vi "MeasureTransconductance.vi"(0 ".NET Refnum in":refnum<k24>, 1 "UiDefinition":T1, 2 "Junction Name":string, 5 ".NET Refnum":refnum<k24>, 7 "appended path":path, 9 "Path":path, 12 "new file path (Not A Path if cancelled)":path, 13 "Function":string) -> (4 "Cluster":cluster{dbl[], dbl[]}, 15 "error out":errorcluster)   [LabVIEW 2020]
uses:
  UIReferences.ctl
  C:/Users/User/Desktop/Automation/CurrentVersion/LabviewDXFViewer/bin/Release/LabviewDXFViewer.exe
  LabviewDXFViewer/bin/Release/LabviewDXFViewer.exe
  <vilib>/Utility/file.llb/Write Delimited Spreadsheet (DBL).vi
  <vilib>/Utility/file.llb/Write Delimited Spreadsheet (string).vi
panel:
  in  "CurrentPositionIndex":i32
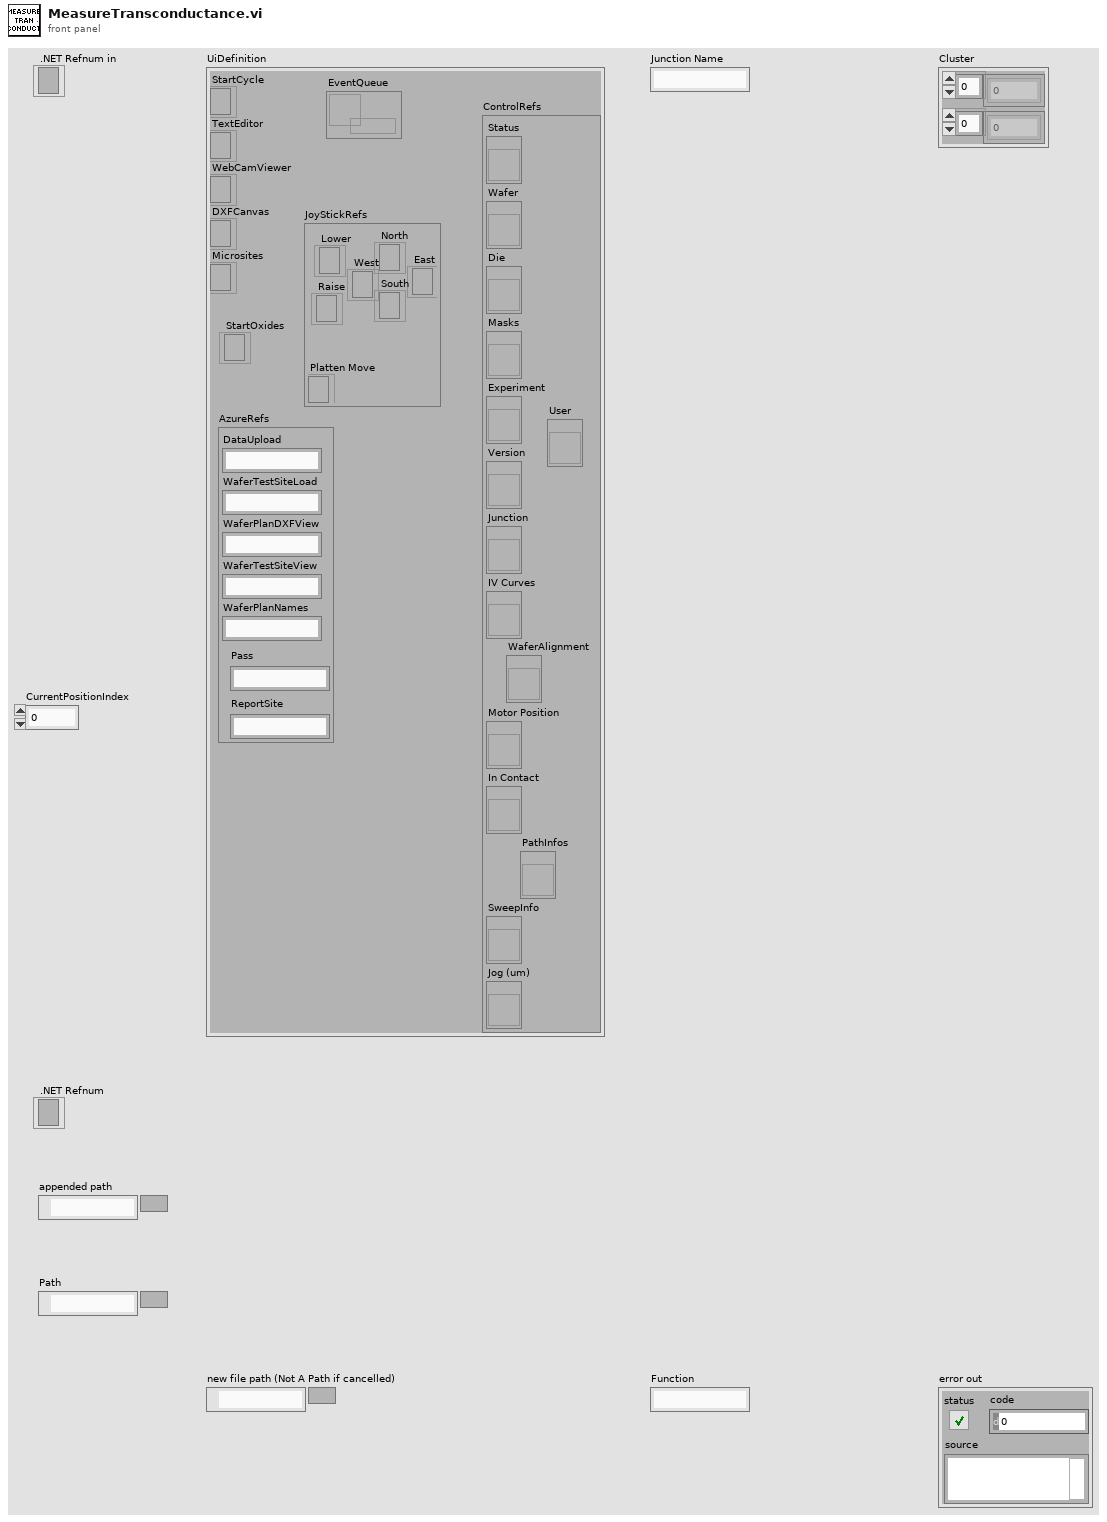
[diagram p1: front panel]
types:
  T1 = typedef "UIReferences.ctl" = cluster{"StartCycle":refnum<k24>, "TextEditor":refnum<k24>, "WebCamViewer":refnum<k24>, "DXFCanvas":refnum<k24>, "Microsites":refnum<k24>, "JoyStickRefs":cluster{"North":refnum<k24>, "Lower":refnum<k24>, "Raise":refnum<k24>, "Platten Move":refnum<k24>, "West":refnum<k24>, "East":refnum<k24>, "South":refnum<k24>}, "AzureRefs":cluster{"DataUpload":string, "WaferTestSiteLoad":string, "WaferPlanDXFView":string, "WaferTestSiteView":string, "WaferPlanNames":string, "Pass":string, "ReportSite":string}, "ControlRefs":cluster{"Status":refnum<vi>, "Wafer":refnum<vi>, "Die":refnum<vi>, "Masks":refnum<vi>, "Experiment":refnum<vi>, "Version":refnum<vi>, "Junction":refnum<vi>, "IV Curves":refnum<vi>, "Motor Position":refnum<vi>, "In Contact":refnum<vi>, "SweepInfo":refnum<vi>, "Jog (um)":refnum<vi>, "PathInfos":refnum<vi>, "User":refnum<vi>, "WaferAlignment":refnum<vi>}, "EventQueue":refnum<queue>, "StartOxides":refnum<k24>}
  T2 = typedef "CapacitanceInfos.ctl" = cluster{"Conductance":dbl, "CapacitanceIV":dbl, "Intercept":dbl, "CapacitanceSW":dbl, "Sum":dbl, "CapacitanceInfos":T3[], "CapacitancePhase":dbl, "dC/dV":dbl, "Function":string, "OtherInfo":dbl[][]}
  T3 = typedef "CapacitanceRecord.ctl" = cluster{"Freq":dbl, "Vpp":dbl, "PhaseS":dbl, "Irms":dbl, "PhaseC":dbl, "Theta":dbl, "VDrive":dbl, "Capacitance":dbl, "Other":dbl}
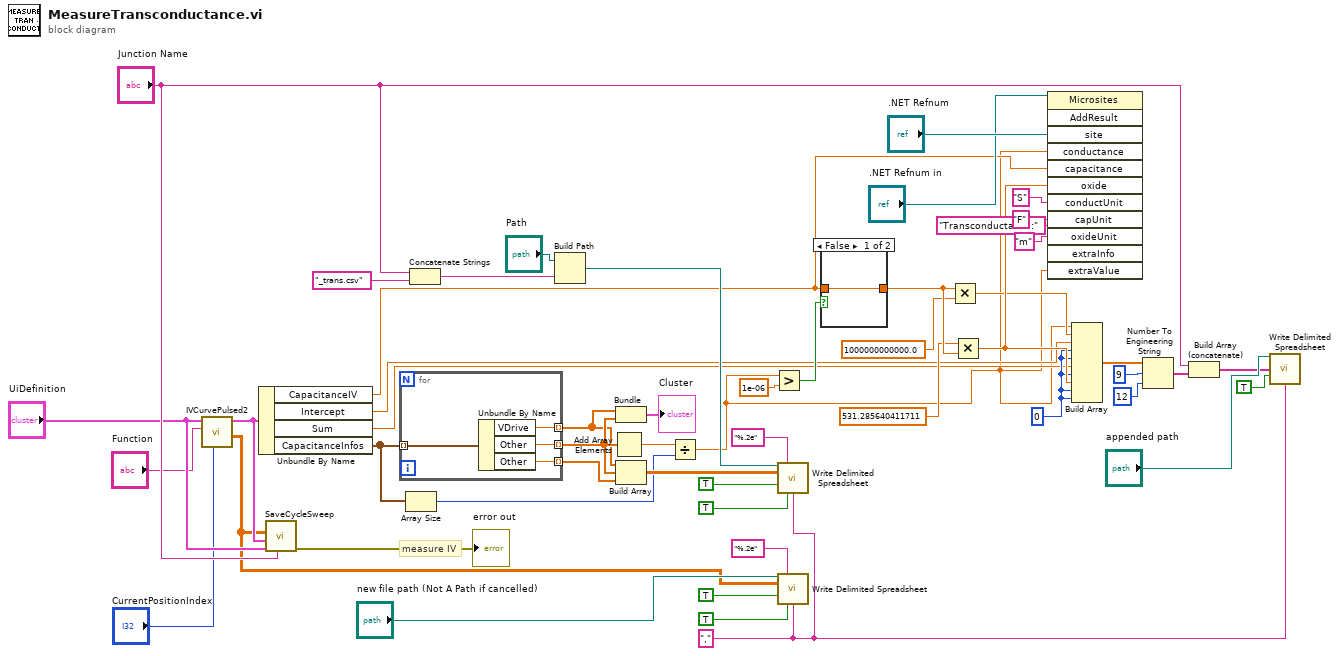
[diagram p0: block diagram]
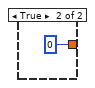
[diagram p2: hidden frame]
diagram:
  w4 = "," ("delimiter (\\t)")
  w26 = 0
  # "measure IV"
  n1 = call "IVCurvePulsed2.vi"("CurrentPositionIndex"="CurrentPositionIndex", "Program"="Function", "UiDefinition"="UiDefinition") -> ("appended array"=w12:dbl[][], "InfoCluster"=w25:T2)  [unwired: 7 in]
  n2 = Unbundle By Name(w25) -> ("CapacitanceIV"=w27:dbl, "Intercept"=w15:dbl, "Sum"=w16:dbl, "CapacitanceInfos"=w36:T3[])
  n3 = call "SaveCycleSweep.vi"("JunctionName"="Junction Name", "UiDefinition 2"="UiDefinition", "InfoCluster"=w25, "appended array"=w12) -> ("error out"=→"error out":errorcluster)  [unwired: 7 in]
  n4 = for {
    tunnel: w36 -> [w56] mode=indexing
    tunnel: [w55] -> w49 mode=indexing
    tunnel: [w54] -> w50 mode=indexing
    tunnel: [w53] -> w51 mode=indexing
    n5 = Unbundle By Name(w56) -> ("VDrive"=w55:dbl, "Other"=w54:dbl, "Other"=w53:dbl)
  }
  n6 = Array Size(array=w36) -> (size(s)=w35:i32)
  n7 = Concatenate Strings("Junction Name", "_trans.csv" ("string")) -> (w42:string)
  n8 = Build Path(base path="Path", name or relative path=w42) -> (appended path=w48:path)
  n9 = Add Array Elements(numeric array=w50) -> (sum=w34:dbl)
  n10 = Bundle(w49, w50) -> (→"Cluster":cluster{dbl[], dbl[]})  [unwired: 1 in]
  n11 = Build Array(w49, w50, w51) -> (w52:dbl[][])
  n12 = Divide(x=w34, y=w35) -> (x/y=w3:dbl)
  n13 = Greater?(x=w3, y=1e-06) -> (0:w19:bool)
  n14 = call-poly <vilib>:"Write Delimited Spreadsheet.vi"("file path (dialog if empty)"=w48, "format (%.3f)"="%.2e", "2D data"=w52, "append to file? (new file:F)"=TRUE, "transpose? (no:F)"=TRUE, "delimiter (\\t)"=w4) -> ()  [unwired: 8 in, 2 out]
  n15 = call-poly <vilib>:"Write Delimited Spreadsheet.vi"("file path (dialog if empty)"="new file path (Not A Path if cancelled)", "format (%.3f)"="%.2e", "2D data"=w12, "append to file? (new file:F)"=TRUE, "transpose? (no:F)"=TRUE, "delimiter (\\t)"=w4) -> ()  [unwired: 8 in, 2 out]
  n16 = case shown="False" w19 {
    tunnel: [w57 0] -> w38
    tunnel: w27 -> [w57 _]
    frame False {
    }
    frame True {
    }
  }
  n17 = Multiply(x=w38, y=1000000000000.0) -> (x*y=w17:dbl)
  n18 = Multiply(x=531.285640411711, y=w38) -> (x*y=w39:dbl)
  n19 = invoke class="Microsites" method="AddResult"(reference=".NET Refnum in", "site"=".NET Refnum", "conductance"=w3, "capacitance"=w27, "oxide"=w39, "conductUnit"="S", "capUnit"="F", "oxideUnit"="m" ("interceptUnit"), "extraInfo"="Transconductance:", "extraValue"=w3) -> ()  [unwired: 2 in, 12 out]
  n20 = Build Array(w3, w17, w15, w26, w26, w16, w26, w39, w26, w26) -> (w14:dbl[])
  n21 = Number To Engineering String(2:i16 12 ("precision (6)"), 3:i16 9 ("width (-)"), 4:w14) -> (0:w6:string[])  [unwired: 1 in]
  n22 = Build Array (concatenate)("Junction Name", w6) -> (w8:string[])
  n23 = call-poly <vilib>:"Write Delimited Spreadsheet.vi"("file path (dialog if empty)"="appended path", "1D data"=w8, "append to file? (new file:F)"=TRUE, "delimiter (\\t)"=w4) -> ()  [unwired: 10 in, 2 out]
